vi "Equi-Ripple HighPass (DBL).vi"(0 "# of taps":i32=32, 1 "stop freq":dbl=0.2 format="%0.2f", 2 "high freq":dbl=0.25 format="%0.2f", 3 "sampling freq: fs":dbl=1.0 format="%0.2f", 5 "X":dbl[](array[numeric])) -> (4 "error":i32, 7 "Filtered X":dbl[](array[numeric]))   [LabVIEW 2010, in "NI_AALBase.lvlib"]
doc: "Generates a highpass FIR filter with equi-ripple characteristics using the Parks-McClellan algorithm and the <B># of taps</B>, <B>stop freq</B>, <B>high freq</B>, and <B>sampling freq: fs</B>. The Equi-Ripple HighPass VI then applies a linear-phase, highpass filter to the input sequence <B>X</B> using the Convolution VI to obtain <B>Filtered X</B>. Wire data to the <B>X</B> input to determine the polymorphic instance to use or manually select the instance."
uses:
  NI_AALBase.lvlib
  1D Convolution (DBL).vi
  NI_AALPro.lvlib
panel:
  # "Equi-Ripple\n Highpass FIR Filter"
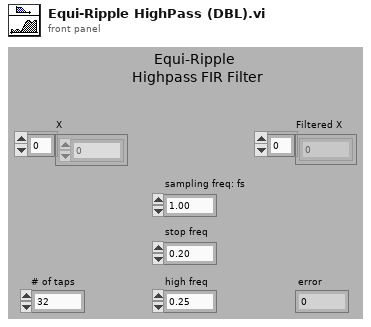
[diagram p1: front panel]
types:
  T1 = cluster{"Amplitude":dbl, "DC":dbl, "stop freq":dbl, "Weight":dbl}
  T2 = cluster{"Amplitude":dbl, "high freq":dbl, dbl, "Weight":dbl}
  T3 = cluster{"Amplitude":dbl, "high freq":dbl, "stop freq":dbl, "Weight":dbl}[]
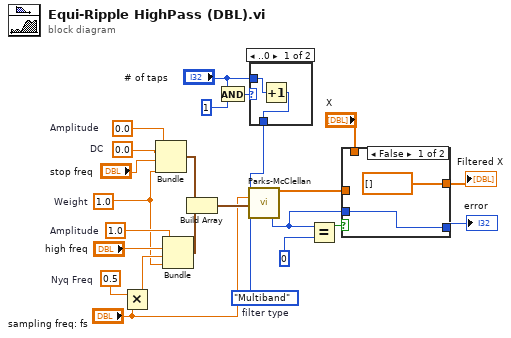
[diagram p0: block diagram]
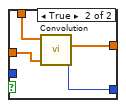
[diagram p3: hidden frame]
diagram:
  w10 = enum32{"Multiband", "Differentiator", "Hilbert"}."Multiband"  # filter type
  w3 = 1.0  # Weight
  w22 = 0.5  # Nyq Freq
  w4 = 1.0  # Amplitude
  w1 = 0.0  # DC
  w2 = 0.0  # Amplitude
  n1 = Multiply(x=w22, y="sampling freq: fs") -> (x*y=w21:dbl)
  n2 = Bundle("Amplitude"=w2, "DC"=w1, "stop freq"="stop freq", "Weight"=w3) -> (w20:T1)  [unwired: 1 in]
  n3 = Bundle("Amplitude"=w4, "high freq"="high freq", w21, "Weight"=w3) -> (w19:T2)  [unwired: 1 in]
  n4 = Build Array(w20, w19) -> (w9:T3)
  n5 = And(x="# of taps", y=1) -> (x .and. y?=w14:i32)
  n6 = case shown="..0" w14 {
    tunnel: "# of taps" -> [w26 w27]
    tunnel: [w25 w27] -> w12
    frame ..0 {
      n7 = Increment(x=w26) -> (x+1=w25:i32)
    }
    frame 1.. {
    }
  }
  n8 = call "Parks-McClellan.vi"("filter type"=w10, "Band Parameters"=w9, "sampling freq: fs"="sampling freq: fs", "# of taps"=w12) -> ("error"=w7:i32, "h"=w11:dbl[])  [unwired: 1 out]
  n9 = Equal?(x=w7, y=0) -> (x = y?=w6:bool)
  n10 = case shown="False" w6 {
    tunnel: w7 -> [w29 _]
    tunnel: [w29 w30] -> w18
    tunnel: [dbl[] [] ("empty array") w31] -> w17
    tunnel: "X" -> [_ w33]
    tunnel: w11 -> [_ w32]
    frame False {
    }
    frame True {
      n11 = call-poly "Convolution.vi"("Y"=w32, "X"=w33) -> ("error"=w30:i32, "X * Y"=w31:dbl[])  [unwired: 8 in]
    }
  }
  "Filtered X" <- w17
  "error" <- w18
